vi "3-lorentzian-heat-response.vi"(0 "zeta":dbl(slide)=0.000285 min=0.0 max=0.3 step=1e-06 scale=0.01..10.0 scale format="%#_3p", 1 "T1":dbl(slide)=0.000285 min=0.0 max=0.3 step=1e-06 scale=0.01..10.0 scale format="%#_3p", 2 "tauS":dbl(slide)=0.000285 min=0.0 max=0.3 step=1e-06 scale=0.01..10.0 scale format="%#_3p", 3 "tauN":dbl(slide)=0.000285 min=0.0 max=0.3 step=1e-06 scale=0.01..10.0 scale format="%#_3p", 4 "tauC":dbl(slide)=0.000285 min=0.0 max=0.3 step=1e-06 scale=0.01..10.0 scale format="%#_3p", 5 "kappa0":dbl(slide)=0.000285 min=0.0 max=0.3 step=1e-06 scale=0.01..10.0 scale format="%#_3p", 7 "omega (rad/sec)":dbl=0.1 format="%#_10f", 8 "action":T1, 9 "m1 IN":dbl=0.1 format="%#_10f", 11 "m2 IN":dbl=0.1 format="%#_10f", 13 "m3 IN":dbl=0.1 format="%#_10f") -> (14 "Romega":cdb=0.1+0.0i format="%#_10f", 15 "m1":dbl=0.1 format="%#_10f", 16 "m2":dbl=0.1 format="%#_10f", 17 "m3":dbl=0.1 format="%#_10f", 18 "String":string)   [LabVIEW 2020]
uses:
  3-lorentzian-heat-response action.ctl
  142dd4c5-f9ed-c64b-bc14-a88e3e2c450a.vi
  <vilib>/Analysis/polynomials.llb/Multiply Polynomials (DBL).vi
  <vilib>/Analysis/polynomials.llb/Polynomial Roots (DBL).vi
  <vilib>/Comparison/Less/Less Functor/Less Functor.lvclass
  <vilib>/Analysis/NI_AALPro.lvlib
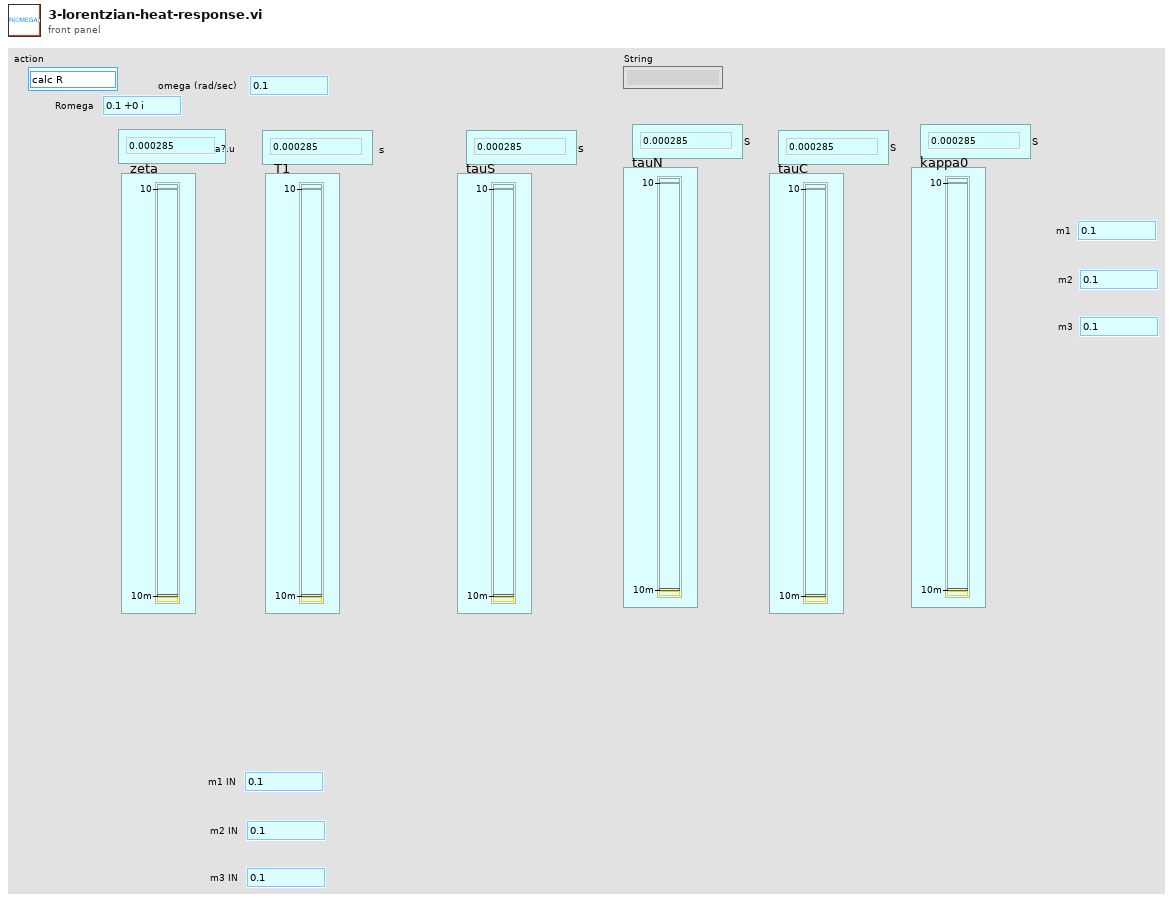
[diagram p1: front panel]
types:
  T1 = typedef "3-lorentzian-heat-response action.ctl" = enum16{"calc R", "create string", "calc m1m2m3", "dζ", "dT1", "dτS", "dτN", "dτC", "d-all", "dκ0", "T(K)", "m1", "m2", "m3", "parse string", "θ (deg)", "B (T)", "onlygrads", "newton", "create emty string"}
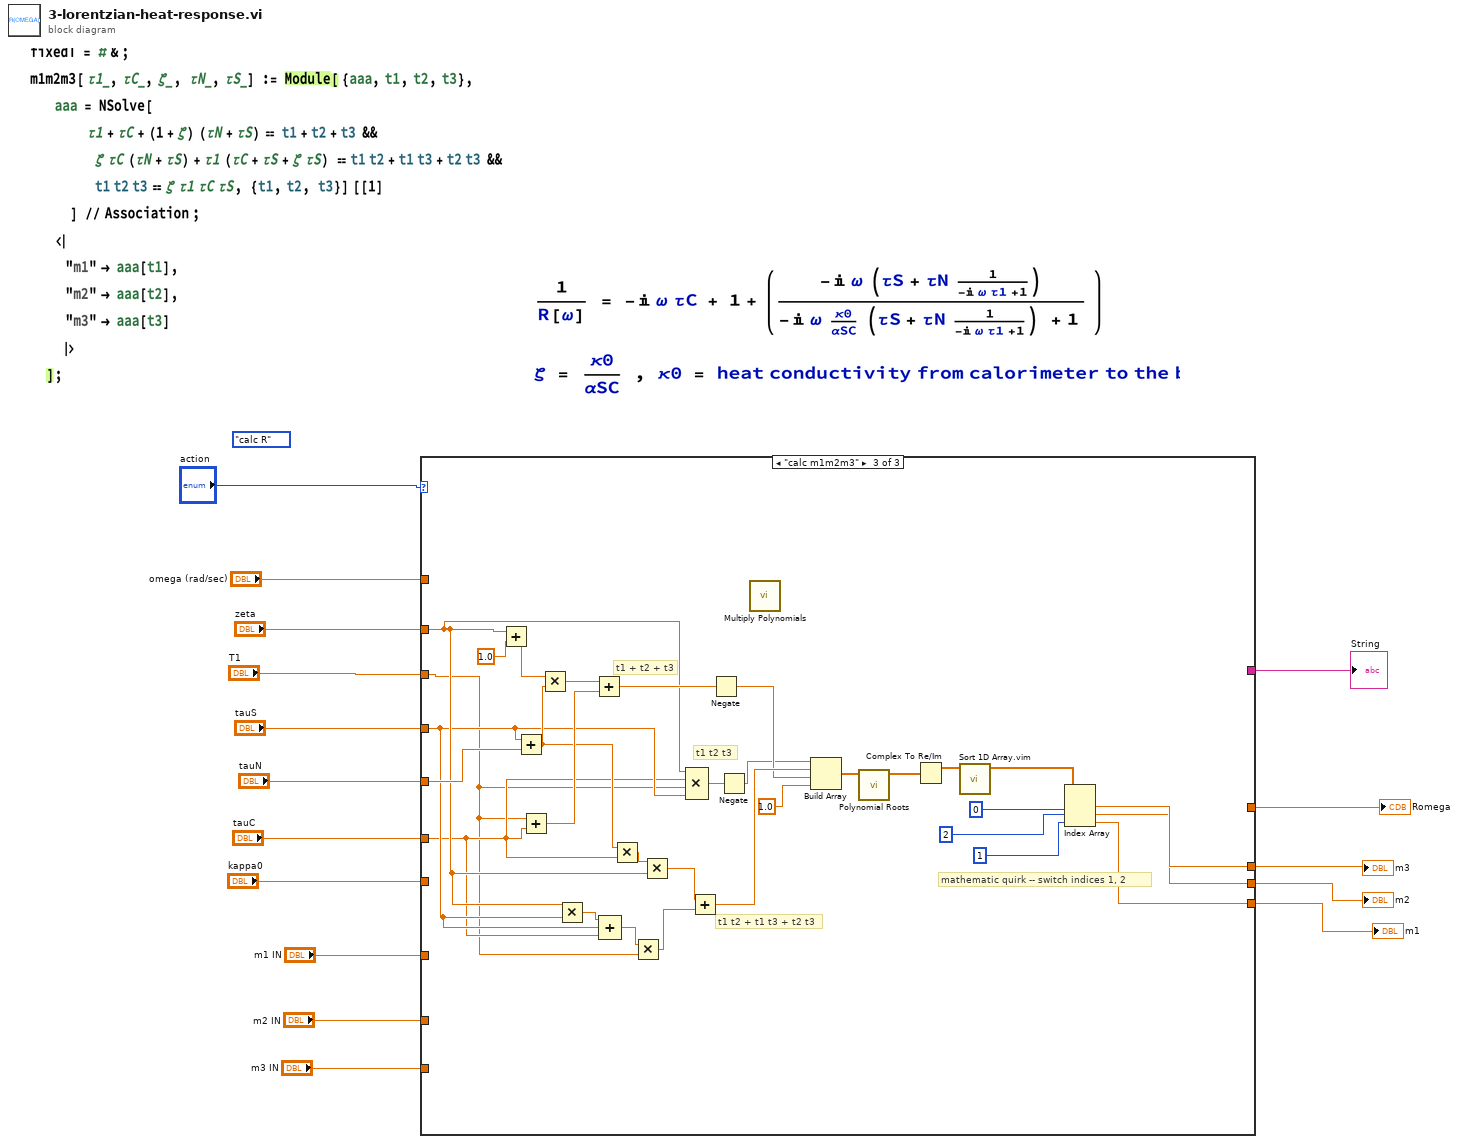
[diagram p0: block diagram]
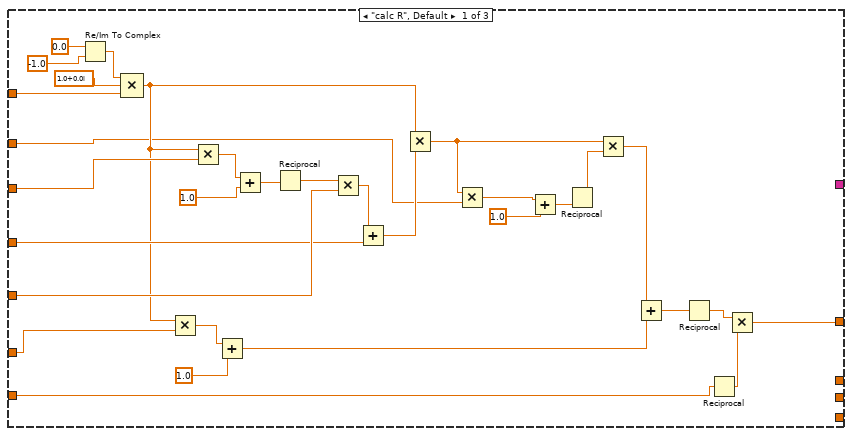
[diagram p2: hidden frame]
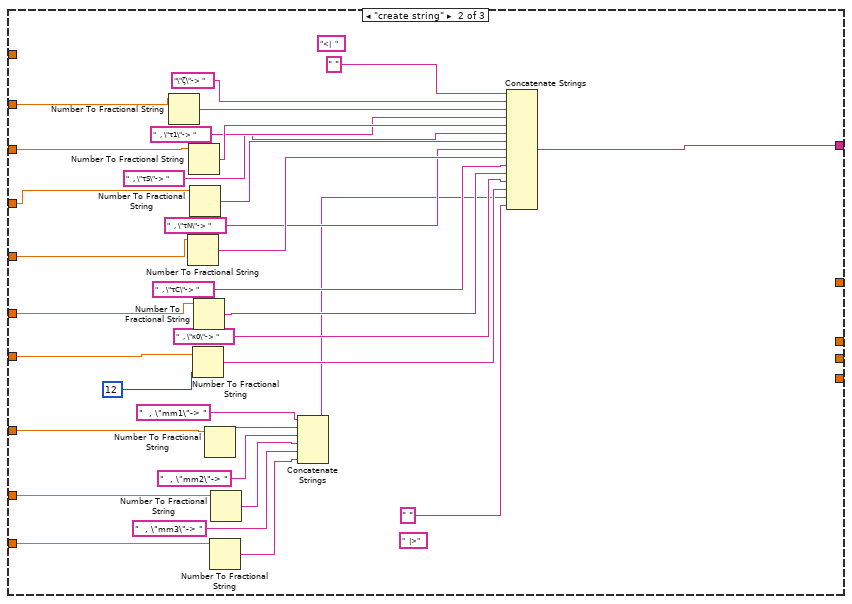
[diagram p3: hidden frame]
diagram:
  (unwired) 3-lorentzian-heat-response_action."calc R" ("action")
  n1 = case shown="\"calc m1m2m3\"" "action" {
    tunnel: "tauC" -> [w33 w77 w96]
    tunnel: "omega (rad/sec)" -> [w36 _ _]
    tunnel: "T1" -> [w35 w78 w94]
    tunnel: "tauN" -> [w41 w70 w109]
    tunnel: "tauS" -> [w39 w71 w97]
    tunnel: "zeta" -> [w29 w79 w99]
    tunnel: [w17 _ _] -> w8
    tunnel: "kappa0" -> [w20 w76 _]
    tunnel: [_ w61 _] -> w7
    tunnel: [_ _ w87] -> w6
    tunnel: [_ _ w83] -> w5
    tunnel: [_ _ w82] -> w4
    tunnel: "m1 IN" -> [_ w59 _]
    tunnel: "m2 IN" -> [_ w58 _]
    tunnel: "m3 IN" -> [_ w57 _]
    frame "calc R", Default {
      n2 = Re/Im To Complex(1:-1.0 ("y"), 2:0.0 ("x")) -> (0:w37:cdb)
      n3 = Compound Arithmetic op=MULTIPLY(w37, cdb 1.0+0.0i ("value"), w36) -> (w31:cdb)
      n4 = Multiply(x=w31, y=w33) -> (x*y=w32:cdb)
      n5 = Multiply(x=w31, y=w35) -> (x*y=w34:cdb)
      n6 = Add(x=w32, y=1.0) -> (x+y=w23:cdb)
      n7 = Add(x=w34, y=1.0) -> (x+y=w43:cdb)
      n8 = Reciprocal(x=w43) -> (1/x=w42:cdb)
      n9 = Multiply(x=w42, y=w41) -> (x*y=w40:cdb)
      n10 = Add(x=w40, y=w39) -> (x+y=w30:cdb)
      n11 = Multiply(x=w31, y=w30) -> (x*y=w25:cdb)
      n12 = Multiply(x=w25, y=w29) -> (x*y=w27:cdb)
      n13 = Add(x=w27, y=1.0) -> (x+y=w26:cdb)
      n14 = Reciprocal(x=w26) -> (1/x=w24:cdb)
      n15 = Multiply(x=w25, y=w24) -> (x*y=w22:cdb)
      n16 = Add(x=w22, y=w23) -> (x+y=w21:cdb)
      n17 = Reciprocal(x=w21) -> (1/x=w19:cdb)
      n18 = Reciprocal(x=w20) -> (1/x=w18:dbl)
      n19 = Multiply(x=w19, y=w18) -> (x*y=w17:cdb)
    }
    frame "create string" {
      (unwired) "<|  "
      (unwired) "  |>"
      n20 = Number To Fractional String(number=w79) -> (F-format string=w75:string)  [unwired: 3 in]
      n21 = Number To Fractional String(number=w70) -> (F-format string=w72:string)  [unwired: 3 in]
      n22 = Number To Fractional String(number=w78) -> (F-format string=w74:string)  [unwired: 3 in]
      n23 = Number To Fractional String(number=w71) -> (F-format string=w73:string)  [unwired: 3 in]
      n24 = Number To Fractional String(number=w76, precision (6)=i16 12 ("width (-)")) -> (F-format string=w62:string)  [unwired: 2 in]
      n25 = Number To Fractional String(number=w77) -> (F-format string=w64:string)  [unwired: 3 in]
      n26 = Number To Fractional String(number=w59) -> (F-format string=w55:string)  [unwired: 3 in]
      n27 = Number To Fractional String(number=w57) -> (F-format string=w51:string)  [unwired: 3 in]
      n28 = Number To Fractional String(number=w58) -> (F-format string=w53:string)  [unwired: 3 in]
      n29 = Concatenate Strings("  , \"mm1\"-> ", w55, "  , \"mm2\"-> ", w53, "  , \"mm3\"-> ", w51) -> (w50:string)
      n30 = Concatenate Strings(" ", "\"ζ\"-> ", w75, "  , \"τ1\"-> ", w74, "  , \"τS\"-> ", w73, "  , \"τN\"-> ", w72, "  , \"τC\"-> ", w64, "  , \"κ0\"-> ", w62, w50, " ") -> (w61:string)
    }
    frame "calc m1m2m3" {
      # "mathematic quirk -- switch indices 1, 2"
      # "t1 t2 + t1 t3 + t2 t3"
      # "t1 + t2 + t3"
      # "t1 t2 t3"
      n31 = Add(x=w99, y=1.0) -> (x+y=w108:dbl)
      n32 = Add(x=w97, y=w109) -> (x+y=w101:dbl)
      n33 = Add(x=w94, y=w96) -> (x+y=w106:dbl)
      n34 = Multiply(x=w108, y=w101) -> (x*y=w107:dbl)
      n35 = Multiply(x=w99, y=w97) -> (x*y=w98:dbl)
      n36 = Add(x=w107, y=w106) -> (x+y=w102:dbl)
      n37 = Compound Arithmetic op=ADD(w98, w97, w96) -> (w95:dbl)
      n38 = Multiply(x=w101, y=w96) -> (x*y=w100:dbl)
      n39 = Multiply(x=w95, y=w94) -> (x*y=w92:dbl)
      n40 = Multiply(x=w100, y=w99) -> (x*y=w93:dbl)
      n41 = Compound Arithmetic op=MULTIPLY(w99, w96, w94, w97) -> (w105:dbl)
      n42 = Add(x=w93, y=w92) -> (x+y=w91:dbl)
      n43 = Negate(x=w102) -> (-x=w81:dbl)
      n44 = Negate(x=w105) -> (-x=w80:dbl)
      n45 = call-poly <vilib>:"Multiply Polynomials.vi"() -> ()  [unwired: 10 in, 2 out]
      n46 = Build Array(w80, w91, w81, 1.0 ("element")) -> (w103:dbl[])
      n47 = call-poly <vilib>:"Polynomial Roots.vi"("P(x)"=w103) -> ("Roots"=w85:cdb[])  [unwired: 9 in, 1 out]
      n48 = Complex To Re/Im(x + iy=w85) -> (x=w84:dbl[])  [unwired: 1 out]
      n49 = call "Sort 1D Array.vim"("unsorted array"=w84) -> ("sorted array"=w86:dbl[])  [unwired: 10 in]
      n50 = Index Array(array=w86, index #1=0 ("index"), index #2=2 ("index"), index #3=1 ("index")) -> (element #1=w87:dbl, element #2=w83:dbl, element #3=w82:dbl)
    }
  }
  "Romega" <- w8
  "String" <- w7
  "m3" <- w6
  "m2" <- w5
  "m1" <- w4
